vi "main.vi"() -> ()   [LabVIEW 2021]
panel:
  out "filenames":string[](array[string])
  in  "Tag":T1(ring)
  in  "image":path
  in  "stop":bool
  out "Image 2":T2(plugin-control)
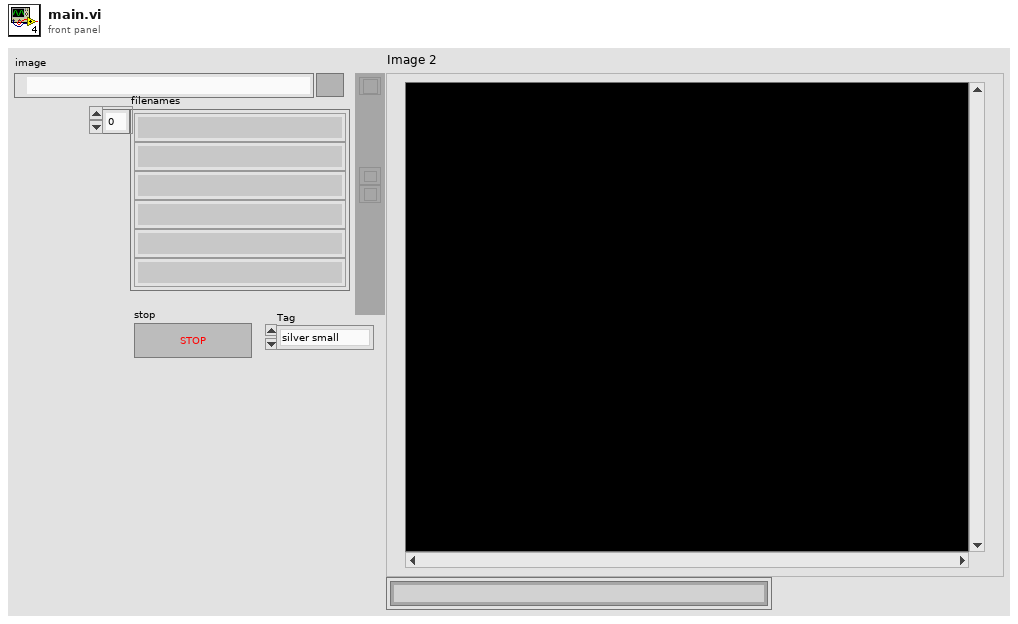
[diagram p1: front panel]
types:
  T1 = enum16{"silver small", "silver medium", "silver huge", "black small", "black medium", "black huge"}
  T2 = typedef "IMAQ Image.ctl" = refnum<image>
  T3 = cluster{"Zoom Tool":bool, "Selection Tool":bool, "Pan Tool":bool, "Point Tool":bool, "Line Tool":bool, "Rectangle Tool":bool, "Rotated Rectangle Tool":bool, "Polyline Tool":bool, "Polygon Tool":bool, "Freehand Tool":bool, "Closed Freehand Tool":bool, "Ellipse Tool":bool, "Annulus Tool":bool}
  T4 = cluster{cluster{i32, i32, i32, i32}, "name":string}[]
  T5 = cluster{"width":string, "height":string, "depth ":string}
  T6 = cluster{"Global Rectangle":i32[], "Contours":cluster{"Contour Type":u32, "ROI Type":u32, "Points":i32[]}[]}
  T7 = cluster{cluster{i32, i32, i32, i32}, "name":string}
  T8 = cluster{"name":string, "pose":string, "truncated":string, "occluded":string, "difficult":string, "bndbox":cluster{"xmin":string, "ymin":string, "xmax ":string, "ymax":string}}[]
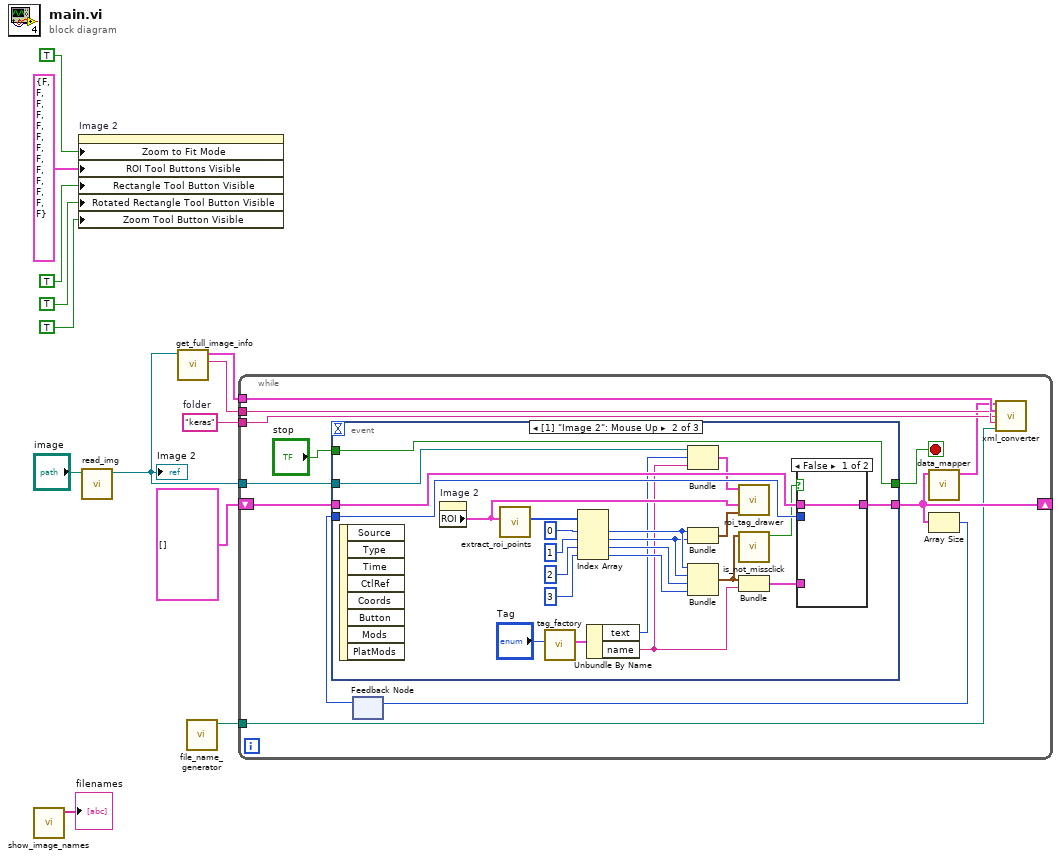
[diagram p0: block diagram]
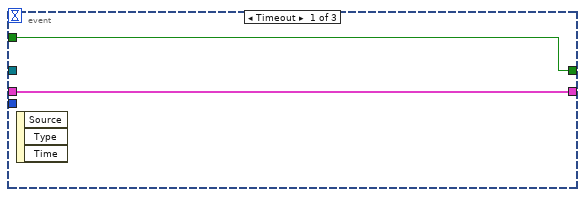
[diagram p2: hidden frame]
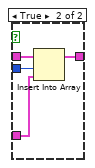
[diagram p3: hidden frame]
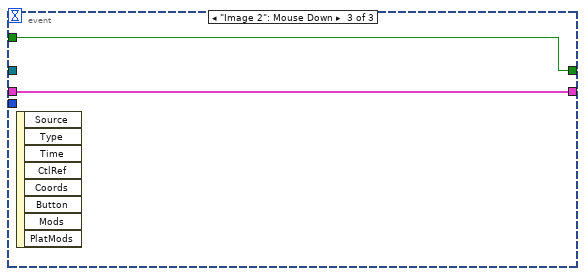
[diagram p4: hidden frame]
diagram:
  w8 = "keras"  # folder
  n1 = call "show_image_names.vi"() -> ("filenames"=→"filenames":string[])  [unwired: 11 in]
  n2 = property on="Image 2" class="ImageControl"("Zoom to Fit Mode"=TRUE, "ROI Tool Buttons Visible"=T3 {"Zoom Tool"=FALSE, "Selection Tool"=FALSE, "Pan Tool"=FALSE, "Point Tool"=FALSE, "Line Tool"=FALSE, "Rectangle Tool"=FALSE, "Rotated Rectangle Tool"=FALSE, "Polyline Tool"=FALSE, "Polygon Tool"=FALSE, "Freehand Tool"=FALSE, "Closed Freehand Tool"=FALSE, "Ellipse Tool"=FALSE, "Annulus Tool"=FALSE} ("ROI Tool Buttons Visible:All Elements"), "Rectangle Tool Button Visible"=TRUE ("Zoom to Fit Mode"), "Rotated Rectangle Tool Button Visible"=TRUE ("ROI Tool Buttons Visible:Rotated Rectangle Tool Button Visible"), "Zoom Tool Button Visible"=TRUE ("ROI Tool Buttons Visible:Zoom Tool Button Visible")) -> ()  [unwired: 2 in, 2 out]
  n3 = call "read_img.vi"("input image 2"="image") -> ("Image 2"=w11:T2)  [unwired: 10 in]
  "Image 2" <- w11
  n4 = call "get_full_image_info.vi"("Image"=w11) -> ("Image Name"=w9:string, "size"=w10:T5)  [unwired: 9 in]
  n5 = call "file_name_generator.vi"() -> ("file_name"=w6:path)  [unwired: 11 in]
  n6 = while {
    tunnel: w11 -> [w25]
    shift-right: [w21] -> _
    shift-left: T4 [] ("array") -> [w22]
    tunnel: w10 -> [w20]
    tunnel: w9 -> [w19]
    tunnel: w8 -> [w18]
    tunnel: w6 -> [w16]
    stop <- w14 stop-if-true
    n7 = feedback #1() -> (w23:i32)  [unwired: 1 in]
    n8 = event shown="[1] \"Image 2\": Mouse Up" {
      selector: _ -> [_ _ _]
      dyn-events: _ -> [_ _ _]
      timeout: _ -> [_ _ _]
      tunnel: w25 -> [_ w32 _]
      tunnel: w22 -> [w27 w40 w58]
      tunnel: [w27 w39 w58] -> w21
      tunnel: w23 -> [_ w38 _]
      tunnel: "stop" -> [w26 w28 w57]
      tunnel: [w26 w28 w57] -> w14
      event Timeout {
        n9 = event-data() -> ()  [unwired: 1 in, 3 out]
      }
      event "Image 2": Mouse Up {
        n10 = event-data() -> ()  [unwired: 1 in, 8 out]
        n11 = property on="Image 2" class="ImageControl"() -> ("ROI"=w35:T6)  [unwired: 2 in, 2 out]
        n12 = call "extract_roi_points.vi"("input cluster"=w35) -> ("Points"=w37:i32[])  [unwired: 10 in]
        n13 = call "tag_factory.vi"("Enum"="Tag") -> ("Cluster"=w49:cluster{"name":string, "text":u32})  [unwired: 10 in]
        n14 = Index Array(array=w37, index #1=0 ("index"), index #2=1 ("index"), index #3=2 ("index"), index #4=3 ("index")) -> (element #1=w45:i32, element #2=w44:i32, element #3=w43:i32, element #4=w42:i32)
        n15 = Unbundle By Name(w49) -> ("text"=w34:u32, "name"=w33:string)
        n16 = Bundle("Image 2"=w32, "text"=w34, "name"=w33) -> (w31:cluster{"Image 2":T2, "text":u32, "name":string})  [unwired: 1 in]
        n17 = Bundle(w45, w44) -> (w36:cluster{i32, i32})  [unwired: 1 in]
        n18 = Bundle(w45, w44, w43, w42) -> (w30:cluster{i32, i32, i32, i32})  [unwired: 1 in]
        n19 = call "roi_tag_drawer.vi"("Origin"=w36, "ROI Descriptor"=w35, "Cluster"=w31) -> ()  [unwired: 9 in]
        n20 = call "is_not_missclick.vi"("input"=w30) -> ("notMissclick"=w29:bool)  [unwired: 10 in]
        n21 = Bundle(w30, "name"=w33) -> (w41:T7)  [unwired: 1 in]
        n22 = case shown="False" w29 {
          tunnel: w41 -> [_ w56]
          tunnel: w40 -> [w52 w55]
          tunnel: [w52 w54] -> w39
          tunnel: w38 -> [_ w53]
          frame False {
          }
          frame True {
            n23 = Insert Into Array(array=w55, index=w53, new element=w56) -> (w54:T4)
          }
        }
      }
      event "Image 2": Mouse Down {
        n24 = event-data() -> ()  [unwired: 1 in, 8 out]
      }
    }
    n25 = call "data_mapper.vi"("input"=w21) -> ("output"=w17:T8)  [unwired: 10 in]
    n26 = Array Size(array=w21) -> (size(s)=w24:i32)
    n27 = feedback-in #1(w24) -> ()
    n28 = call "xml_converter.vi"("object"=w17, "size"=w20, "folder"=w18, "filename"=w19, "XML File Path 2"=w16) -> ()  [unwired: 11 in]
  }
